vi "ReadLCRsettings.vi"(5 "error in (no error)":errorcluster, 6 "LCRControl in":refnum<class "LCRControl.lvclass">) -> (0 "error out":errorcluster, 1 "RC Configuration":u16(ring) items=["serial", "parallel"], 2 "AC frequency [Hz]":i32, 3 "LCRControl out":refnum<class "LCRControl.lvclass">, 4 "AC amplitude [V]":sgl)   [LabVIEW 2018, in "LCRControl.lvclass"]
uses:
  LCRControl.lvclass
  LCRControl.lvclass/LCRControl.ctl
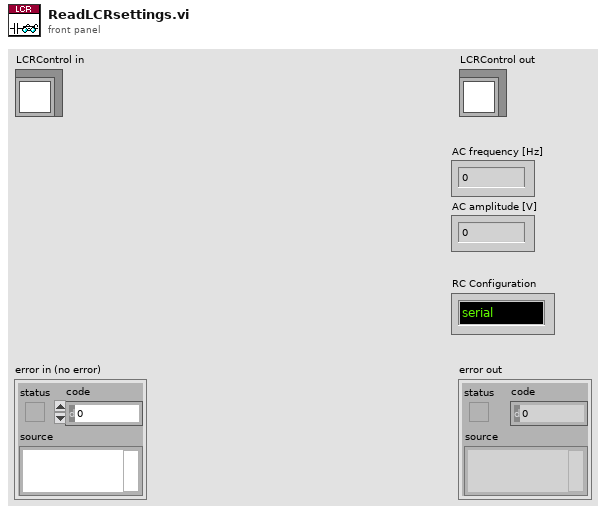
[diagram p1: front panel]
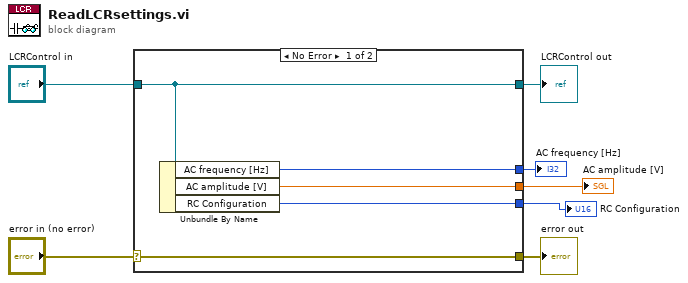
[diagram p0: block diagram]
diagram:
  n1 = case shown="No Error" "error in (no error)" {
    selector: "error in (no error)" -> [w12 w13]
    tunnel: [w12 w13] -> w6
    tunnel: [w11 w14] -> w4
    tunnel: "LCRControl in" -> [w11 w14]
    tunnel: [w10 _] -> w3
    tunnel: [w9 _] -> w2
    tunnel: [w8 _] -> w1
    frame No Error {
      n2 = Unbundle By Name(w11) -> ("AC frequency [Hz]"=w10:i32, "AC amplitude [V]"=w9:sgl, "RC Configuration"=w8:u16)
    }
    frame Error {
    }
  }
  "error out" <- w6
  "LCRControl out" <- w4
  "AC frequency [Hz]" <- w3
  "AC amplitude [V]" <- w2
  "RC Configuration" <- w1
